vi "Read Attributes.vi"(11 "Abstract Message Template in":refnum<class "Abstract Message Template.lvclass">) -> (2 "Payload":cluster{})   [LabVIEW 2020, in "Abstract Message Template.lvclass"]
uses:
  Abstract Message Template.lvclass
  Abstract Message Template.lvclass/Abstract Message Template.ctl
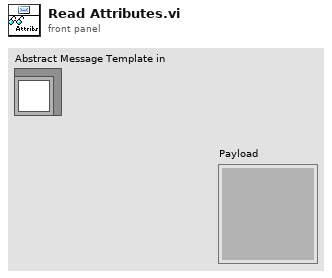
[diagram p1: front panel]
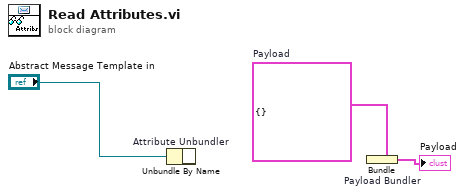
[diagram p0: block diagram]
diagram:
  w1 = cluster{} {}  # Payload
  n1 = Unbundle By Name "Attribute Unbundler"("Abstract Message Template in") -> ()  [unwired: 1 out]
  n2 = Bundle "Payload Bundler"(cluster=w1) -> (→"Payload":cluster{"Boolean":void})  [unwired: 1 in]
